vi "Gyro calib routine.vi"(6 "Connection Status":T1={"MAC Address"="", "cnx handle"=0, "cnx flags"=0, "Address Type"=125, "Connection Interval (ms)"=125, "Timeout(ms)"=125, "Latency"=0, "bonding handle"=0} {"Address Type" items=["Public", "Random"]}, 8 "Error In":errorcluster={"status"=FALSE, "code"=1073676294, "source"="VISA Read in ble_read_message.vi->ble_read_specific_message.vi->ble_evt_attclient_attribute_value.vi->ble_read_by_handle.vi->MPU panel.vi"}, 11 "VISA resource in":refnum<visa-resource-name>="COM50") -> ()   [LabVIEW 2016]
uses:
  <vilib>/BLE/type_def/connection_status_bundle.ctl
  <vilib>/BLE/type_def/address_type.ctl
  Typedef/Gyro calib - States.ctl
  Typedef/BLE char handle.ctl
  Typedef/Gyro FSR.ctl
  <vilib>/Analysis/baseanly.llb/Mean (DBL).vi
  <vilib>/BLE/ble_functions/ble_write_by_handle_uint8array.vi
  <vilib>/Analysis/NI_AALBase.lvlib
panel:
  in  "Set & Save":bool
  in  "Exit":bool
  in  "Next":bool
  out "Calibration results":i32(listbox)=-1
  out "Instructions":string="Press START CALIBRATION to calibrate the gyroscope."
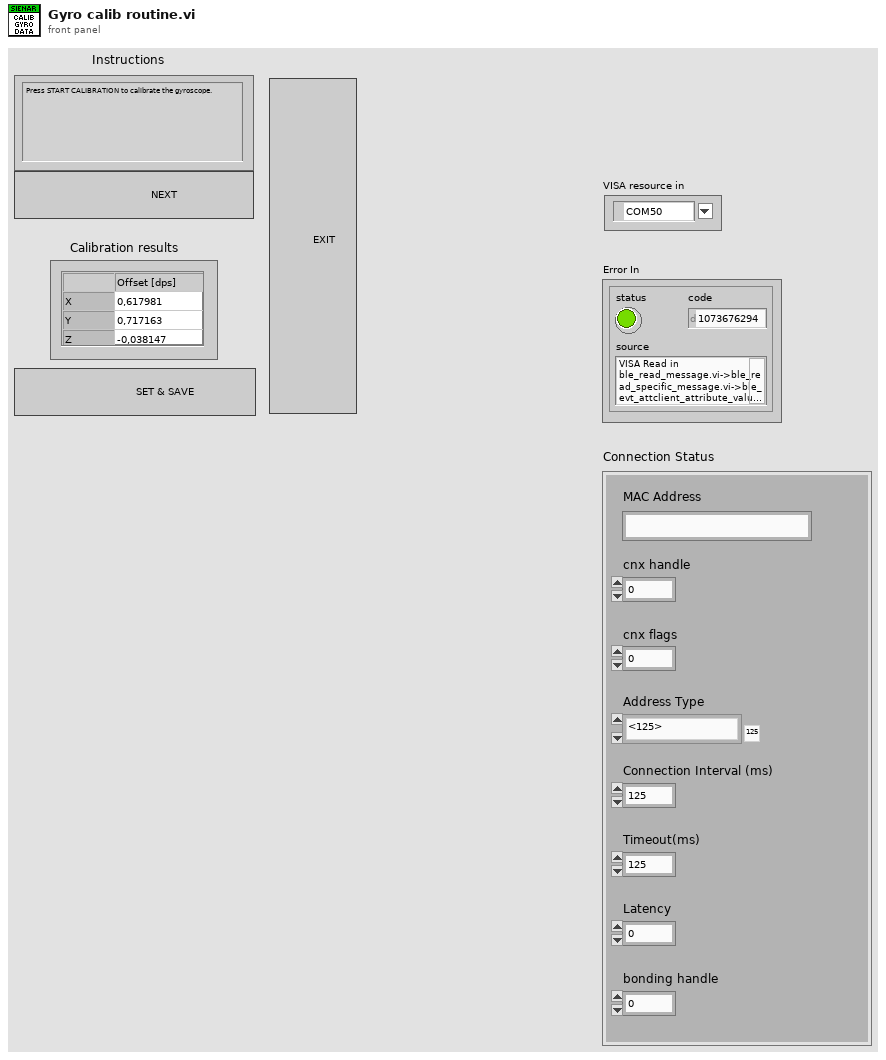
[diagram p1: front panel]
types:
  T1 = typedef "connection_status_bundle.ctl" = cluster{"MAC Address":string, "cnx handle":u8, "cnx flags":u8, "Address Type":T2, "Connection Interval (ms)":u16, "Timeout(ms)":u16, "Latency":u16, "bonding handle":u8}
  T2 = typedef "address_type.ctl" = u8
  T3 = typedef "Gyro calib - States.ctl" = enum16{"Start calibration", "Acquire Offset", "Display results", "Set & Save", "Exit"}
  T4 = typedef "Gyro FSR.ctl" = enum16{"±250dps", "±500dps", "±1000dps", "±2000dps"}
  T5 = enum16{"Accelerometer", "Gyroscope", "Magnetometer"}
  T6 = typedef "BLE char handle.ctl" = u16
  T7 = cluster{"AccelData":cluster{"AccelX":i16, "AccelY":i16, "AccelZ":i16}, "GyroData":cluster{"GyroX":i16, "GyroY":i16, "GyroZ":i16}, "MagData":cluster{"MagX":i16, "MagY":i16, "MagZ":i16}}
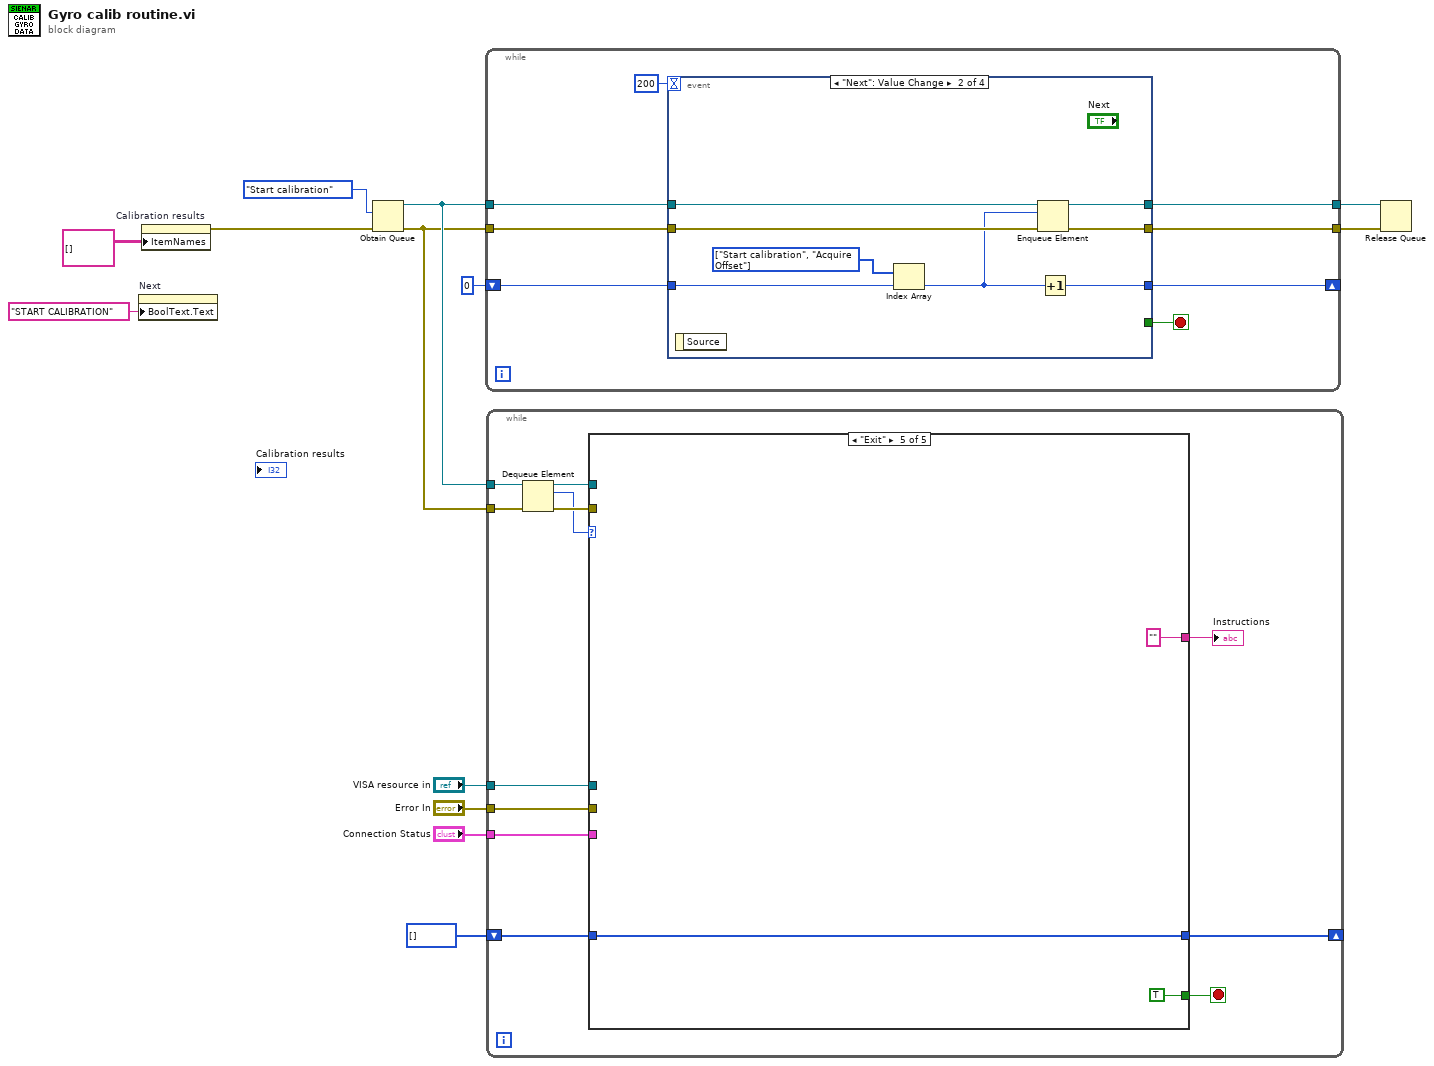
[diagram p0: block diagram]
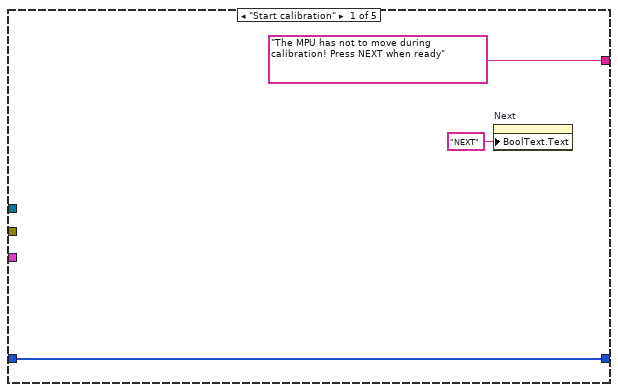
[diagram p2: hidden frame]
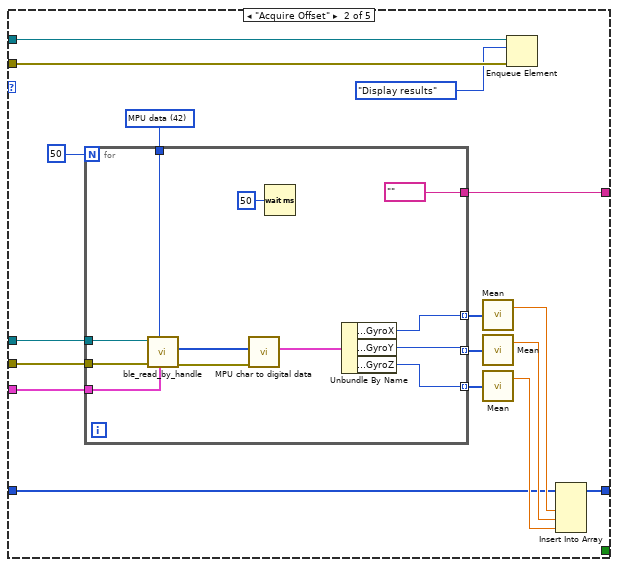
[diagram p3: hidden frame]
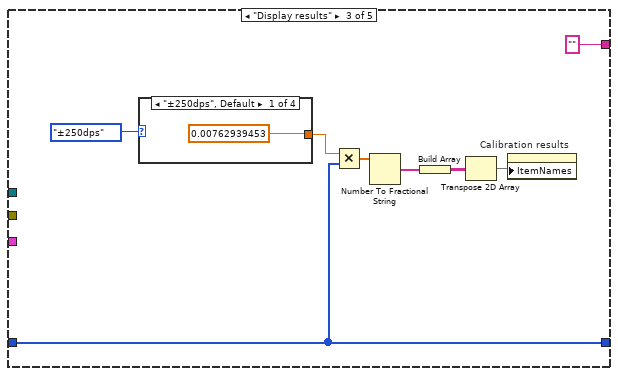
[diagram p4: hidden frame]
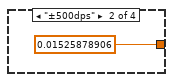
[diagram p5: hidden frame]
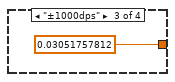
[diagram p6: hidden frame]
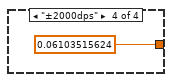
[diagram p7: hidden frame]
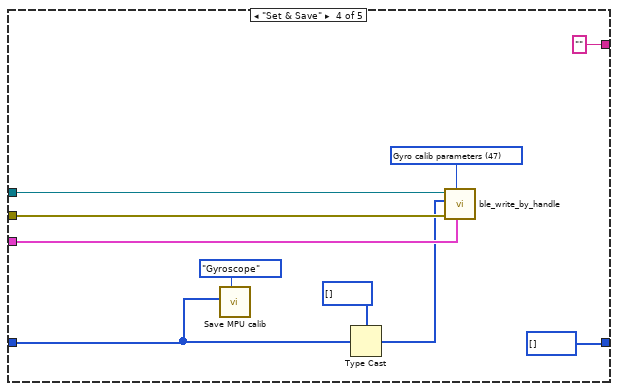
[diagram p8: hidden frame]
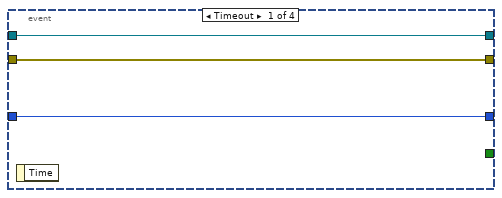
[diagram p9: hidden frame]
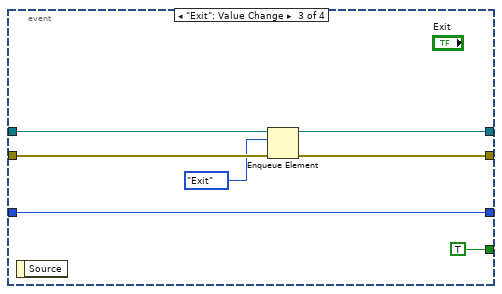
[diagram p10: hidden frame]
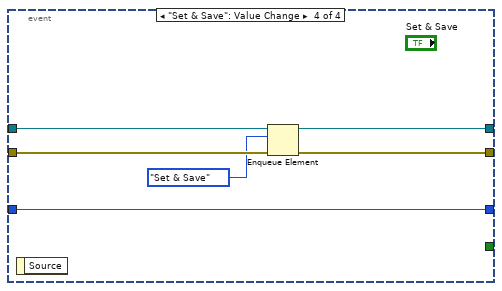
[diagram p11: hidden frame]
diagram:
  n1 = property on="Next" class="Bool"("BoolText.Text"="START CALIBRATION" ("Boolean Text.Text")) -> ()  [unwired: 2 in, 2 out]
  n2 = property on="Calibration results" class="MCListbox (strict)"("ItemNames"=string[][] [] ("Item Names")) -> (error out=w3:errorcluster)  [unwired: 2 in, 1 out]
  n3 = Obtain Queue(element data type=Gyro_calib_-_States."Start calibration" ("Gyro calib states"), error in (no error)=w3) -> (queue out=w10:refnum<queue>, error out=w9:errorcluster)  [unwired: 3 in, 1 out]
  n4 = while {
    tunnel: w10 -> [w20]
    tunnel: w9 -> [w19]
    tunnel: [w18] -> w13
    tunnel: [w17] -> w12
    shift-right: [w15] -> _
    shift-left: 0 -> [w16]
    stop <- w14 stop-if-true
    n5 = event shown="[1] \"Next\": Value Change" {
      selector: _ -> [_ _ _ _]
      dyn-events: _ -> [_ _ _ _]
      timeout: 200 -> [_ _ _ _]
      tunnel: w20 -> [w24 w32 w39 w45]
      tunnel: w19 -> [w23 w31 w38 w44]
      tunnel: [w24 w30 w36 w41] -> w18
      tunnel: [w23 w29 w37 w42] -> w17
      tunnel: w16 -> [w22 w28 w35 w43]
      tunnel: [w22 w27 w35 w43] -> w15
      tunnel: [_ _ TRUE _] -> w14
      event Timeout {
        n6 = event-data() -> ()  [unwired: 1 in, 1 out]
      }
      event "Next": Value Change {
        w26 = T3[] [enum."Start calibration", enum."Acquire Offset"] items=["Start calibration", "Acquire Offset", "Display results", "Set & Save", "Exit"]
        n7 = event-data() -> ()  [unwired: 1 in, 1 out]
        n8 = Index Array(array=w26, index=w28) -> (element=w25:T3)
        n9 = Enqueue Element(queue=w32, element=w25, error in (no error)=w31) -> (queue out=w30:refnum<queue>, error out=w29:errorcluster)  [unwired: 1 in, 1 out]
        n10 = Increment(x=w25) -> (x+1=w27:T3)
      }
      event "Exit": Value Change {
        n11 = event-data() -> ()  [unwired: 1 in, 1 out]
        n12 = Enqueue Element(queue=w39, element=Gyro_calib_-_States."Exit", error in (no error)=w38) -> (queue out=w36:refnum<queue>, error out=w37:errorcluster)  [unwired: 1 in, 1 out]
      }
      event "Set & Save": Value Change {
        n13 = event-data() -> ()  [unwired: 1 in, 1 out]
        n14 = Enqueue Element(queue=w45, element=Gyro_calib_-_States."Set & Save" ("Gyro calib states"), error in (no error)=w44) -> (queue out=w41:refnum<queue>, error out=w42:errorcluster)  [unwired: 1 in, 1 out]
      }
    }
  }
  n15 = while {
    tunnel: w10 -> [w57]
    tunnel: w9 -> [w56]
    tunnel: "VISA resource in" -> [w52]
    tunnel: "Error In" -> [w51]
    tunnel: "Connection Status" -> [w50]
    shift-right: [w46] -> _
    shift-left: i16[] [] -> [w47]
    stop <- w49 stop-if-true
    n16 = Dequeue Element(queue=w57, error in (no error)=w56) -> (queue out=w55:refnum<queue>, element=w48:T3, error out=w54:errorcluster)  [unwired: 1 in, 1 out]
    n17 = case shown="\"Exit\"" w48 {
      tunnel: w55 -> [_ w66 _ _ _]
      tunnel: w54 -> [_ w65 _ _ _]
      tunnel: ["The MPU has not to move during calibration! Press NEXT when ready" ("message") w72 "" ("message") "" ("message") "" ("message")] -> w53
      tunnel: w52 -> [_ w75 _ w109 _]
      tunnel: w51 -> [_ w74 _ w108 _]
      tunnel: w50 -> [_ w73 _ w107 _]
      tunnel: [_ _ _ _ TRUE] -> w49
      tunnel: w47 -> [w58 w63 w93 w103 w112]
      tunnel: [w58 w62 w93 i16[] [] w112] -> w46
      frame "Start calibration" {
        n18 = property on="Next" class="Bool"("BoolText.Text"="NEXT" ("Boolean Text.Text")) -> ()  [unwired: 2 in, 2 out]
      }
      frame "Acquire Offset" {
        w61 = T6 42 items=["MPU data"=42, "MPU data - DESCR"=43, "Accel calib parameters"=45, "Gyro calib parameters"=47, "Mag calib parameters - 1"=49, "Mag calib parameters - 2"=51, "YPR"=53, "YPR - DESCR"=54, "Strain sensors"=56, "Strain sensors - DESCR"=57, "Wristband"=59, "Wristband - DESCR"=60] ("BLE char handle")
        n19 = for {
          N: 50 -> [_]
          tunnel: [w83] -> w76 mode=indexing
          tunnel: w61 -> [w88]
          tunnel: w75 -> [w87]
          tunnel: w74 -> [w86]
          tunnel: w73 -> [w85]
          tunnel: ["" ("message")] -> w72
          tunnel: [w82] -> w70 mode=indexing
          tunnel: [w81] -> w69 mode=indexing
          n20 = call <vilib>:"ble_read_by_handle.vi"("Connection Status"=w85, "Handle"=w88, "error in (no error)"=w86, "COM Bluegiga in"=w87) -> ("error out"=w80:errorcluster, "characteristic value"=w79:u8[])  [unwired: 5 in, 1 out]
          n21 = call "MPU char to digital data.vi"("Error In"=w80, "MPU characteristic data"=w79) -> ("Digital MPU data"=w78:T7)  [unwired: 8 in, 1 out]
          n22 = Wait (ms)(milliseconds to wait=u32 50) -> ()  [unwired: 1 out]
          n23 = Unbundle By Name(w78) -> ("GyroData.GyroX"=w83:i16, "GyroData.GyroY"=w82:i16, "GyroData.GyroZ"=w81:i16)
        }
        n24 = call-poly <vilib>:"Mean.vi"("X"=w76) -> ("mean"=w71:dbl)  [unwired: 1 out]
        n25 = call-poly <vilib>:"Mean.vi"("X"=w70) -> ("mean"=w68:dbl)  [unwired: 1 out]
        n26 = call-poly <vilib>:"Mean.vi"("X"=w69) -> ("mean"=w67:dbl)  [unwired: 1 out]
        n27 = Enqueue Element(queue=w66, element=Gyro_calib_-_States."Display results", error in (no error)=w65) -> ()  [unwired: 1 in, 3 out]
        n28 = Insert Into Array(array=w63, new element #1=w71, new element #2=w68, new element #3=w67) -> (w62:i16[])  [unwired: 1 in]
      }
      frame "Display results" {
        n29 = case shown="\"±250dps\", Default" Gyro_FSR."±250dps" ("Gyro FSR") {
          tunnel: [0.00762939453 0.01525878906 0.03051757812 0.06103515624] -> w94
          frame "±250dps", Default {
          }
          frame "±500dps" {
          }
          frame "±1000dps" {
          }
          frame "±2000dps" {
          }
        }
        n30 = Multiply(x=w94, y=w93) -> (x*y=w92:dbl[])
        n31 = Number To Fractional String(number=w92) -> (F-format string=w96:string[])  [unwired: 3 in]
        n32 = Build Array(w96) -> (w91:string[][])
        n33 = Transpose 2D Array(2D array=w91) -> (transposed array=w90:string[][])
        n34 = property on="Calibration results" class="MCListbox (strict)"("ItemNames"=w90) -> ()  [unwired: 2 in, 2 out]
      }
      frame "Set & Save" {
        w102 = T6 47 items=["MPU data"=42, "MPU data - DESCR"=43, "Accel calib parameters"=45, "Gyro calib parameters"=47, "Mag calib parameters - 1"=49, "Mag calib parameters - 2"=51, "YPR"=53, "YPR - DESCR"=54, "Strain sensors"=56, "Strain sensors - DESCR"=57, "Wristband"=59, "Wristband - DESCR"=60] ("BLE char handle")
        n35 = call "Save MPU calib.vi"("Calib data type"=T5."Gyroscope", "Calib data"=w103) -> ()  [unwired: 9 in, 1 out]
        n36 = Type Cast(type=u8[] [], x=w103) -> (*(type *) &x=w105:u8[])
        n37 = call-poly <vilib>:"ble_write_by_handle.vi"("Connection Status"=w107, "Handle"=w102, "error in (no error)"=w108, "data (uint8array)"=w105, "COM Bluegiga in"=w109) -> ()  [unwired: 5 in, 2 out]
      }
      frame "Exit" {
      }
    }
    "Instructions" <- w53
  }
  n38 = Release Queue(queue=w13, error in (no error)=w12) -> ()  [unwired: 1 in, 3 out]
